vi "Test Messages.vi"() -> ()   [LabVIEW 2025]
uses:
  LabView/Communication Handle/API/Commands.ctl
  LabView/Communication Handle/API/Expected messages.ctl
panel:
  out "Tx":T1(array[cluster]) {"DATA[0]" format="%.0x"}
  out "Expected messages":T2[](array[typedef]) {"DATA[0]" format="%.0x"; "DATA[1]" format="%.0x"; "DATA[2]" format="%.0x"; "DATA[3]" format="%.0x"}
  in  "input 1":T3=enum."MCU Reset"
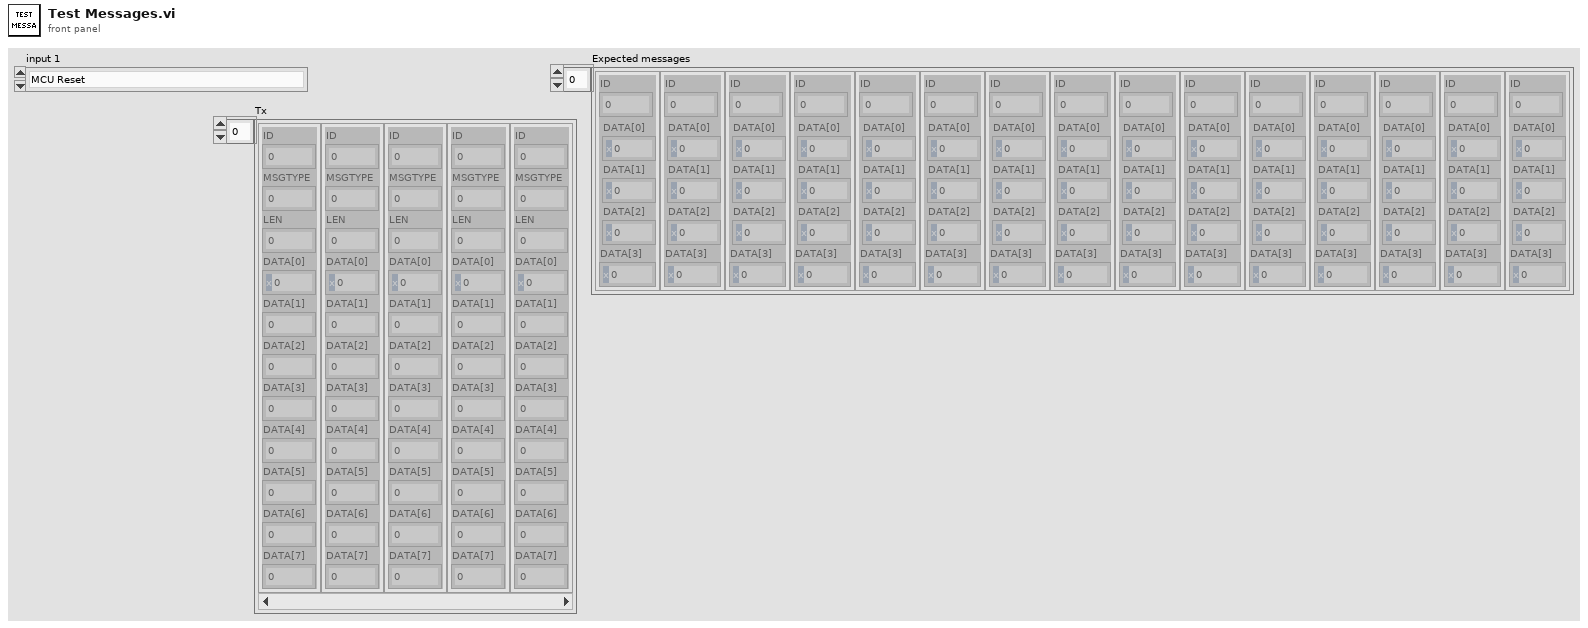
[diagram p1: front panel]
types:
  T1 = cluster{"ID":u32, "MSGTYPE":u8, "LEN":u8, "DATA[0]":u8, "DATA[1]":u8, "DATA[2]":u8, "DATA[3]":u8, "DATA[4]":u8, "DATA[5]":u8, "DATA[6]":u8, "DATA[7]":u8}[]
  T2 = typedef "Expected messages.ctl" = cluster{"DATA[0]":u8, "DATA[1]":u8, "DATA[2]":u8, "DATA[3]":u8, "ID":u32}
  T3 = typedef "Commands.ctl" = enum16{"Nexteer connect", "Write Polarity", "Write BEMF", "Write Torque Scale Sensors T1", "Write Torque Scale Sensors T2", "Trim HW Torque Sensors T1", "Trim HW Torque Sensors T2", "Read HW Torque Trim Performed Sensors T1", "Read HW Torque Trim Performed Sensors T2", "Write EOL Offset values to defaults", "Write EOL Gain values to defaults", "Write Serial Number", "Write Hardware Part Number", "Write EPS Serial Number", "Read MEC Counter", "MCU Reset", "Read System State", "Read First Motor Position", "Manufacturing Diagnostic Defeat", "Perform Current Offset ", "Current Offset Status", "Enable Engine Run", "Perform Current Gain ", "Current Gain Status", "Disable Torque Ramp Down ", "Disable Engine Run", "Set Vehicle Speed Override", "Read Offset Values Using FD F5", "Read Gain Values Using FD F4", "Clear Nexteer NTCs", "Read Second Motor Position", "Read ECU Software ID", "Read Internal Software Version", "Read Bootloader ID", "Read Bootloader Software Version", "Read Calibration Release 0", "Read Calibration Release 1", "Read Calibration Release 2", "Read Temperature  ", "Battery Voltage  ", "Read Motor Angle 0", "Read Motor Angle 1 ", "Set Motor Torque Command ", "Read Motor Current   ", "Stop Motor Torque Command", "Read NTCs", "Read Serial Number", "Read HW Part Number", "Read Polarity", "Set NVM Access Defeat", "Read Software Release", "Read Software Build Date", "Write Single Inverter Hardware value", "Write Dual Inverter Hardware value", "Read Single Inverter HW Value", "Read Dual Inverter HW Value", "Write MEC Counter FE", "Write MEC Counter FF", "Read BEMF", "Read Torque 1 FDB6", "Read Torque 2 FDB7", "Read Torque Trim 1 FDB4", "Read Torque Trim 2 FDB5", "Write Torque Trim 1 FDB4", "Write Torque Trim 2 FDB5", "XCP connect", "Read HW Torque T1", "Read HW Torque T2", "Read Motor Speed "}
  T4 = map{string, cluster{"Tx und Rx":cluster{"ID":u32, "MSGTYPE":u8, "LEN":u8, "DATA[0]":u8, "DATA[1]":u8, "DATA[2]":u8, "DATA[3]":u8, "DATA[4]":u8, "DATA[5]":u8, "DATA[6]":u8, "DATA[7]":u8}[], "NoMessges":i32[]}}
  T5 = cluster{"Tx und Rx":cluster{"ID":u32, "MSGTYPE":u8, "LEN":u8, "DATA[0]":u8, "DATA[1]":u8, "DATA[2]":u8, "DATA[3]":u8, "DATA[4]":u8, "DATA[5]":u8, "DATA[6]":u8, "DATA[7]":u8}[], "NoMessges":i32[]}
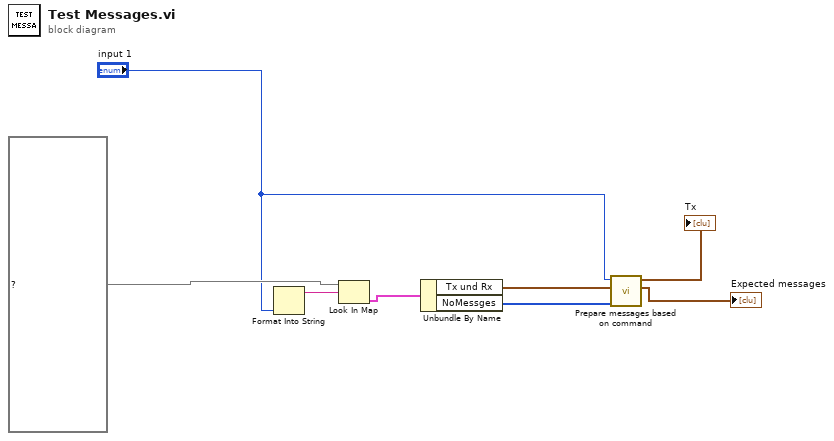
[diagram p0: block diagram]
diagram:
  n1 = Format Into String("input 1") -> (resulting string=w8:string)  [unwired: 3 in, 1 out]
  n2 = Look In Map(map=T4 data[6328B] ("Map"), key=w8) -> (value=w6:T5)  [unwired: 1 in, 1 out]
  n3 = Unbundle By Name(w6) -> ("Tx und Rx"=w5:T1, "NoMessges"=w4:i32[])
  n4 = call "Prepare messages based on command.vi"("NoMessges"=w4, "Tx und Rx"=w5, "Commands"="input 1") -> ("Expected messages"=→"Expected messages":T2[], "Tx"=→"Tx":T1)  [unwired: 7 in]
